vi "G#SubTemplateG3_GetClassAttributesToModify.vi"(0 "reference in":refnum<class "G#SubTemplateG3.lvclass">, 3 "timeout in ms (-1)":i32=-1, 5 "error in (no error)":errorcluster) -> (14 "reference out":refnum<class "G#SubTemplateG3.lvclass">, 15 "class attributes ref":T3, 16 "class attributes":T1, 17 "timeout":bool, 18 "created new":bool, 19 "error out":errorcluster)   [LabVIEW 2020, in "G#SubTemplateG3.lvclass"]
doc: "This VI returns the attributes associated with this class or subclass object reference and places a lock on the object.\n\nIf the object is currently locked for modification by another method, 'Timeout' specifies how long the VI should wait to receive access to the object. The default value waits until the object becomes available.\n\nYou must use this class SetModifiedAttributes VI to set the object's data and release the lock."
uses:
  G#SubTemplateG3.lvclass
  ClassAttributesRef.ctl
  protected/ClassAttributes.ctl
  G#BaseTemplateG3/protected/ClassAttributes.ctl
  G#SubTemplateG3.lvclass/G#SubTemplateG3.ctl
  G#BaseTemplateG3/G#BaseTemplateG3.lvclass
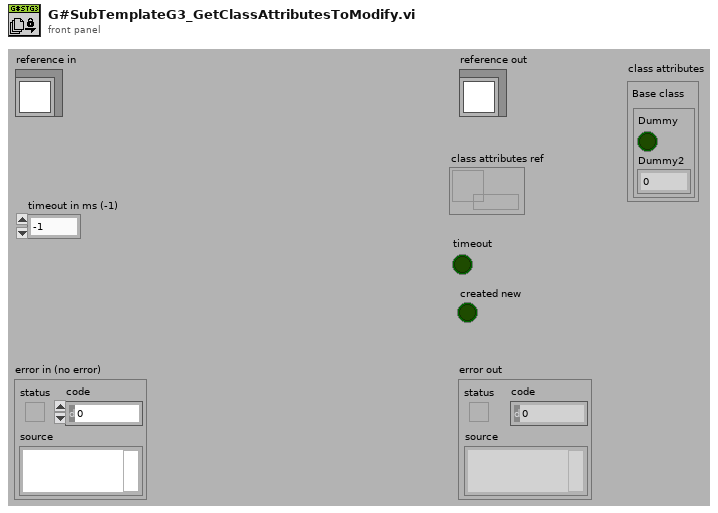
[diagram p1: front panel]
types:
  T1 = typedef "G#SubTemplateG3.lvclass/ClassAttributes.ctl" = cluster{"Base class":T2}
  T2 = typedef "G#BaseTemplateG3.lvclass/ClassAttributes.ctl" = cluster{"Dummy":bool, "Dummy2":dbl}
  T3 = typedef "G#SubTemplateG3.lvclass/ClassAttributesRef.ctl" = refnum<data-value>
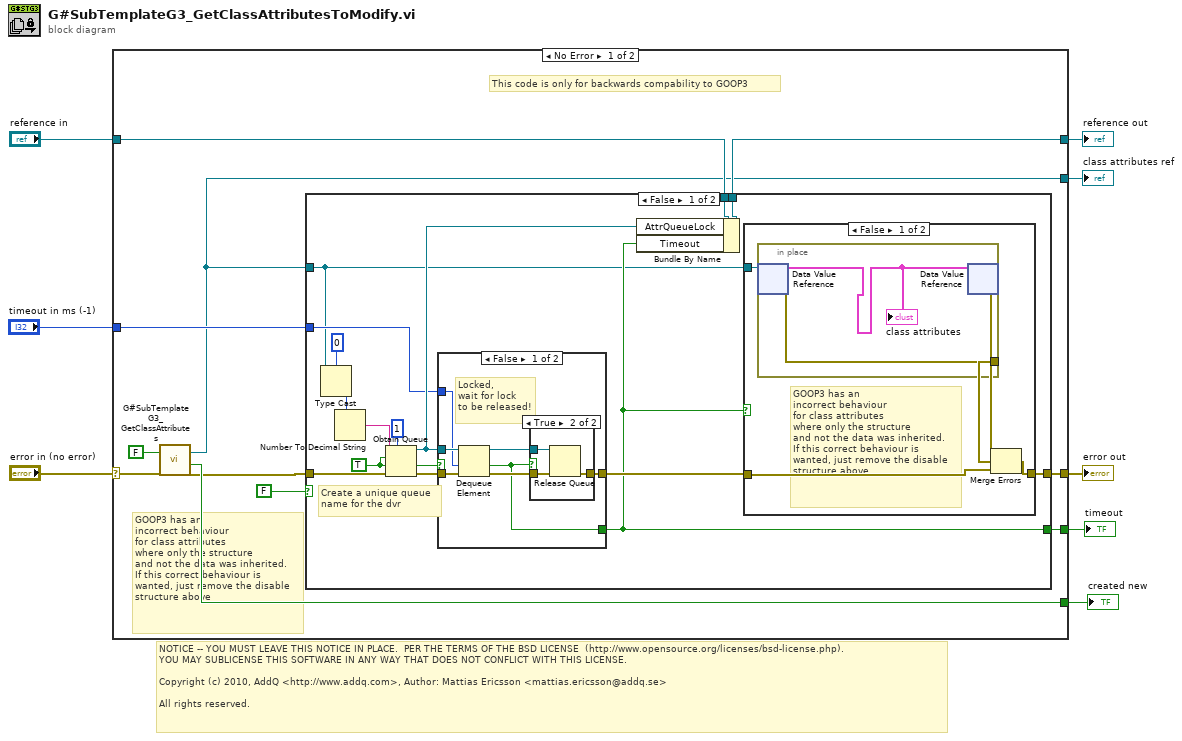
[diagram p0: block diagram]
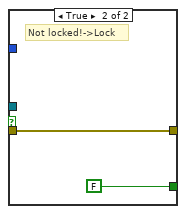
[diagram p3: hidden frame]
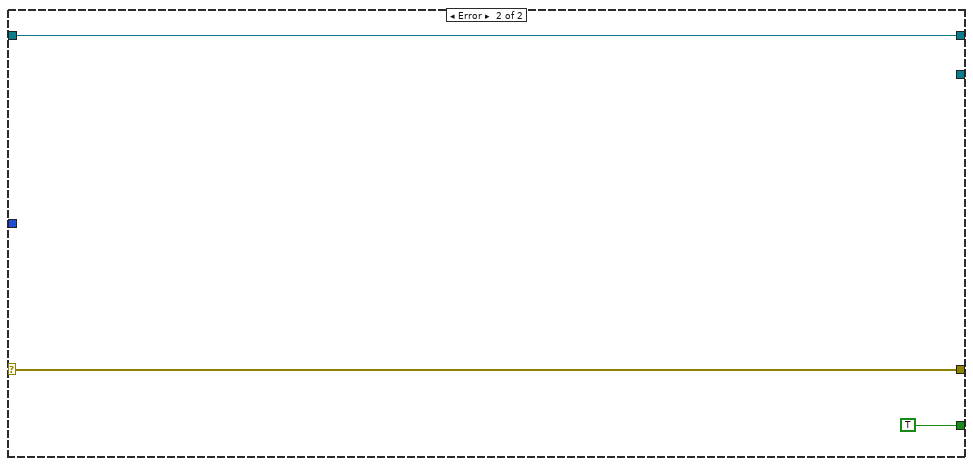
[diagram p6: hidden frame]
diagram:
  # "NOTICE -- YOU MUST LEAVE THIS NOTICE IN PLACE.  PER THE TERMS OF THE BSD LICENSE  (http://www.opensource.org/licenses/bsd-license.php).\nYOU MAY SUBLICENSE THIS SOFTWARE IN ANY WAY THAT DOES NOT CONFLICT WITH THIS LICENSE.\n\nCopyright (c) 2010, AddQ <http://www.addq.com>, Author: Mattias Ericsson <mattias.ericsson@addq.se>\n\nAll rights reserved."
  n1 = case shown="No Error" "error in (no error)" {
    selector: "error in (no error)" -> [w9 w62]
    tunnel: [w19 w62] -> w7
    tunnel: [w15 w61] -> w5
    tunnel: "reference in" -> [w17 w61]
    tunnel: [w12 _] -> w4
    tunnel: "timeout in ms (-1)" -> [w16 _]
    tunnel: [w14 TRUE ("status")] -> w2
    tunnel: [w11 _] -> w1
    frame No Error {
      # "GOOP3 has an\nincorrect behaviour\nfor class attributes\nwhere only the structure\nand not the data was inherited.\nIf this correct behaviour is\nwanted, just remove the disable\nstructure above"
      # "This code is only for backwards compability to GOOP3"
      n2 = call "G#SubTemplateG3_GetClassAttributes.vi"("return data? (T)"=FALSE ("return data"), "error in (no error)"=w9) -> ("class attributes ref"=w12:T3, "created new"=w11:bool, "error out"=w10:errorcluster)  [unwired: 13 in, 2 out]
      n3 = case shown="False" FALSE ("timeout") {
        selector: FALSE ("timeout") -> [_ w58]
        tunnel: [w35 w57] -> w19
        tunnel: w10 -> [w27 w57]
        tunnel: w17 -> [w24 w59]
        tunnel: w16 -> [w23 _]
        tunnel: [w22 w59] -> w15
        tunnel: [w21 w58] -> w14
        tunnel: w12 -> [w20 _]
        frame False {
          w33 = TRUE ("create if not found? (T)")
          # "Create a unique queue\nname for the dvr"
          n4 = Type Cast(type=u32 0, x=w20) -> (*(type *) &x=w26:u32)
          n5 = Number To Decimal String(number=w26) -> (decimal integer string=w34:string)  [unwired: 1 in]
          n6 = Obtain Queue(max queue size (-1, unlimited)=1, name (unnamed)=w34, element data type=w33, create if not found? (T)=w33, error in (no error)=w27) -> (queue out=w28:refnum<queue>, created new?=w30:bool, error out=w31:errorcluster)
          n7 = case shown="False" w30 {
            tunnel: w31 -> [w40 w47]
            tunnel: [w39 w47] -> w29
            tunnel: w28 -> [w42 _]
            tunnel: w23 -> [w41 _]
            tunnel: [w36 FALSE ("status")] -> w21
            frame False {
              # "Locked,\nwait for lock\nto be released!"
              n8 = Dequeue Element(queue=w42, timeout in ms (-1)=w41, error in (no error)=w40) -> (queue out=w37:refnum<queue>, timed out?=w36:bool, error out=w38:errorcluster)  [unwired: 1 out]
              n9 = case shown="True" w36 {
                tunnel: [w43 w46] -> w39
                tunnel: w38 -> [w43 w45]
                tunnel: w37 -> [_ w44]
                frame False {
                }
                frame True {
                  n10 = Release Queue(queue=w44, error in (no error)=w45) -> (error out=w46:errorcluster)  [unwired: 1 in, 2 out]
                }
              }
            }
            frame True {
              # "Not locked!->Lock"
            }
          }
          n11 = Bundle By Name(cluster=w24, "AttrQueueLock"=w28, "Timeout"=w21) -> (w22:refnum<class "G#SubTemplateG3.lvclass">)
          n12 = case shown="False" w21 {
            tunnel: w20 -> [w53 _]
            tunnel: w29 -> [w52 w56]
            tunnel: [w49 w56] -> w35
            frame False {
              # "GOOP3 has an\nincorrect behaviour\nfor class attributes\nwhere only the structure\nand not the data was inherited.\nIf this correct behaviour is\nwanted, just remove the disable\nstructure above"
              n13 = in-place {
                in-place-border: [w54] -> w51
                n14 = in-place-dvr #1(w53) -> (w55:T1, w54:errorcluster)
                "class attributes" <- w55
                n15 = in-place-dvr #1(w55) -> (w50:errorcluster)  [unwired: 1 out]
              }
              n16 = Merge Errors(w50, w51, w52) -> (w49:errorcluster)
            }
            frame True {
              # "Timeout"
            }
          }
        }
        frame True {
        }
      }
    }
    frame Error {
    }
  }
  "error out" <- w7
  "reference out" <- w5
  "class attributes ref" <- w4
  "timeout" <- w2
  "created new" <- w1
